vi "zad9.vi"(8 "error in (no error)":errorcluster, 9 "X":dbl[](array[numeric]), 10 "Parametry":T1, 11 "Ring":u16(ring) items=["Cotangens"=3, "Tangens"=2, "Cosinus"=1, "Sinus"=0]) -> (0 "error out":errorcluster, 2 "Array":dbl[](array[numeric]))   [LabVIEW 2017]
uses:
  <vilib>/express/express arith-compare/Formula/XNode/ExpressFormulaBlockNode.xnode
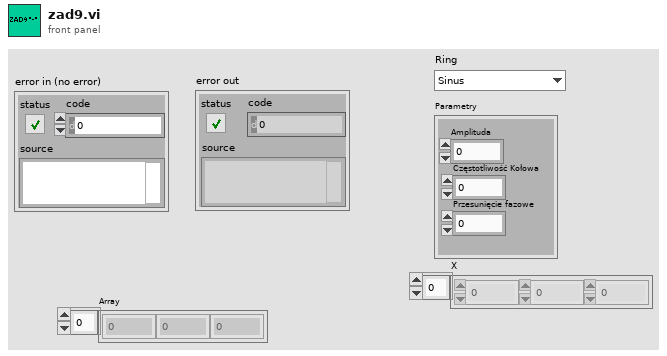
[diagram p1: front panel]
types:
  T1 = cluster{"Amplituda":dbl, "Częstotliwość Kołowa":dbl, "Przesunięcie fazowe":dbl}
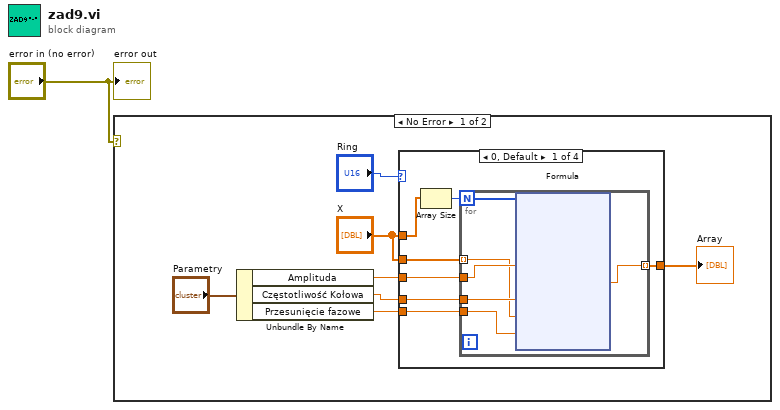
[diagram p0: block diagram]
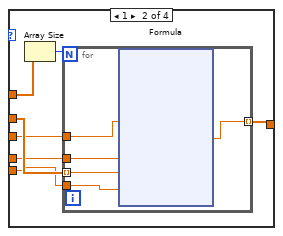
[diagram p2: hidden frame]
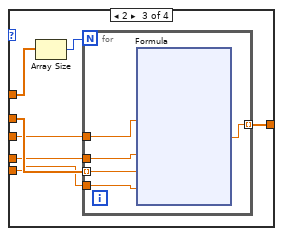
[diagram p3: hidden frame]
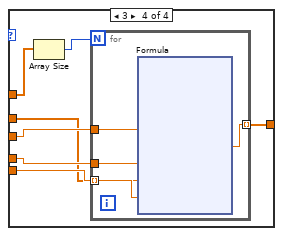
[diagram p4: hidden frame]
diagram:
  n1 = case shown="No Error" "error in (no error)" {
    frame No Error {
      n2 = Unbundle By Name("Parametry") -> ("Amplituda"=w6:dbl, "Częstotliwość Kołowa"=w5:dbl, "Przesunięcie fazowe"=w4:dbl)
      n3 = case shown="0, Default" "Ring" {
        tunnel: "X" -> [w14 w40 w67 w93]
        tunnel: w6 -> [w13 w37 w64 w91]
        tunnel: w5 -> [w12 w36 w63 w90]
        tunnel: w4 -> [w11 w35 w62 w89]
        tunnel: "X" -> [w10 w38 w65 w88]
        tunnel: [w9 w41 w61 w87] -> w2
        frame 0, Default {
          n4 = Array Size(array=w14) -> (size(s)=w15:i32)
          n5 = for {
            N: w15 -> [_]
            tunnel: w13 -> [w20]
            tunnel: w12 -> [w19]
            tunnel: w11 -> [w18]
            tunnel: w10 -> [w17] mode=indexing
            tunnel: [w16] -> w9 mode=indexing
            n6 = xnode "Formula"("A"=w20, "W"=w19, "X"=w17, "0"=w18) -> ("Result"=w16:dbl)  [unwired: 1 in, 1 out]
          }
        }
        frame 1 {
          n7 = Array Size(array=w40) -> (size(s)=w39:i32)
          n8 = for {
            N: w39 -> [_]
            tunnel: [w46] -> w41 mode=indexing
            tunnel: w38 -> [w45] mode=indexing
            tunnel: w37 -> [w44]
            tunnel: w36 -> [w43]
            tunnel: w35 -> [w42]
            n9 = xnode "Formula"("A"=w44, "W"=w43, "X"=w45, "0"=w42) -> ("Result"=w46:dbl)  [unwired: 1 in, 1 out]
          }
        }
        frame 2 {
          n10 = Array Size(array=w67) -> (size(s)=w66:i32)
          n11 = for {
            N: w66 -> [_]
            tunnel: w65 -> [w72] mode=indexing
            tunnel: w64 -> [w71]
            tunnel: w63 -> [w70]
            tunnel: w62 -> [w69]
            tunnel: [w68] -> w61 mode=indexing
            n12 = xnode "Formula"("A"=w71, "W"=w70, "X"=w72, "0"=w69) -> ("Result"=w68:dbl)  [unwired: 1 in, 1 out]
          }
        }
        frame 3 {
          n13 = Array Size(array=w93) -> (size(s)=w92:i32)
          n14 = for {
            N: w92 -> [_]
            tunnel: w91 -> [w98]
            tunnel: w90 -> [w97]
            tunnel: w89 -> [w96]
            tunnel: w88 -> [w95] mode=indexing
            tunnel: [w94] -> w87 mode=indexing
            n15 = xnode "Formula"("A"=w98, "W"=w97, "X"=w95, "0"=w96) -> ("Result"=w94:dbl)  [unwired: 1 in, 1 out]
          }
        }
      }
      "Array" <- w2
    }
    frame Error {
    }
  }
  "error out" <- "error in (no error)"
